vi "Matlab Param Array to Matlab String Array.vi"(8 "error in":errorcluster, 11 "Matlab Param Array":cluster{"Name":string, "Data":variant}[](array[cluster])) -> (0 "error out":errorcluster, 3 "Matlab Strings":string[](array[string]))   [LabVIEW 2012, in "Matlab API.lvlib"]
uses:
  Matlab API.lvlib
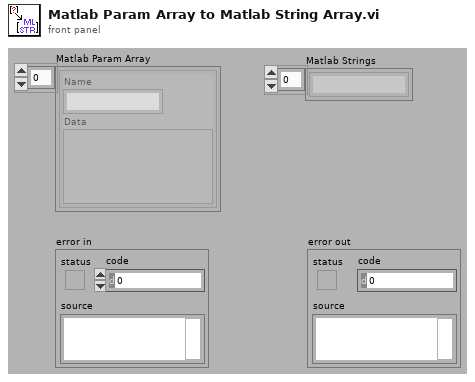
[diagram p1: front panel]
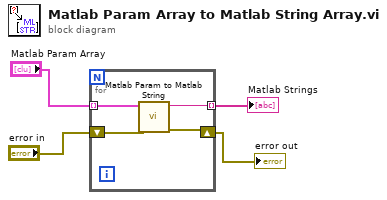
[diagram p0: block diagram]
diagram:
  n1 = for {
    tunnel: "Matlab Param Array" -> [w8] mode=indexing
    shift-right: [w6] -> w1
    shift-left: "error in" -> [w7]
    tunnel: [w5] -> w2 mode=indexing
    n2 = call "Matlab Param to Matlab String.vi"("error in"=w7, "Input Parameter"=w8) -> ("error out"=w6:errorcluster, "Matlab string"=w5:string)  [unwired: 8 out]
  }
  "Matlab Strings" <- w2
  "error out" <- w1
